vi "xps_panel_DO_connect_to_controller.vi"(8 "error in (no error)":errorcluster, 10 "Login Info":T1={"IP Address"="192.168.0.254", "User"="Administrator", "Password"="Administrator"}, 11 "newport_xps_panel in":refnum<class "newport_xps_panel.lvclass">) -> (0 "error out":errorcluster, 3 "newport_xps_panel out":refnum<class "newport_xps_panel.lvclass">)   [LabVIEW 2015, in "newport_xps_panel.lvclass"]
uses:
  newport_xps_panel.lvclass
  xps_login_info.ctl
  newport_xps/newport_xps.lvclass
  newport_xps/newport_xps.lvclass/newport_xps.ctl
  UI/panel_class/panel.lvclass
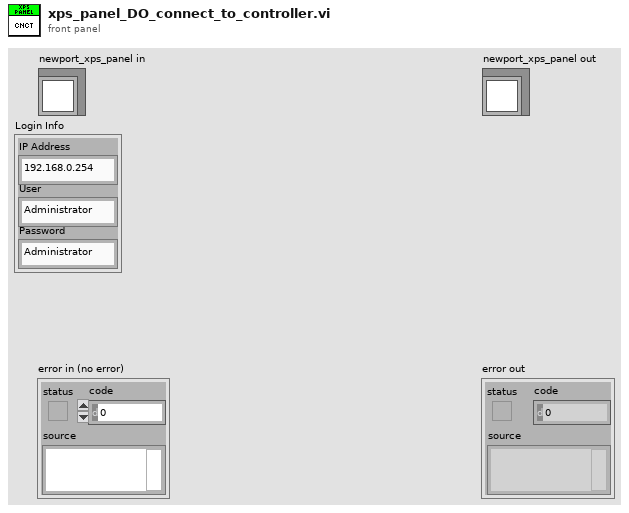
[diagram p1: front panel]
types:
  T1 = typedef "xps_login_info.ctl" = cluster{"IP Address":string, "User":string, "Password":string}
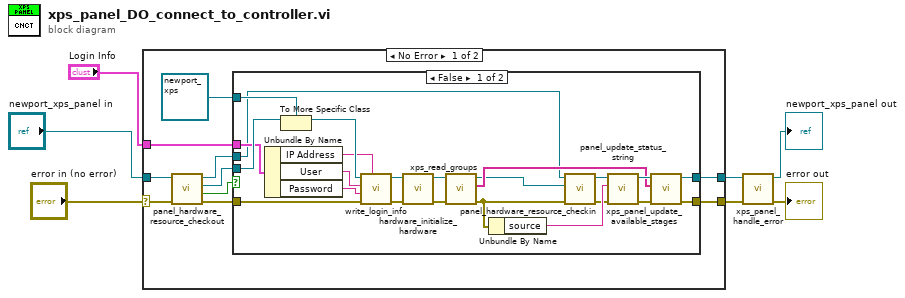
[diagram p0: block diagram]
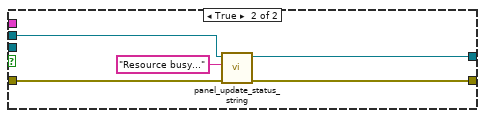
[diagram p2: hidden frame]
diagram:
  n1 = case shown="No Error" "error in (no error)" {
    selector: "error in (no error)" -> [w17 w47]
    tunnel: [w9 w47] -> w4
    tunnel: [w8 w46] -> w2
    tunnel: "newport_xps_panel in" -> [w16 w46]
    tunnel: "Login Info" -> [w10 _]
    frame No Error {
      n2 = call "panel_hardware_resource_checkout.vi"("error in (no error)"=w17, "panel in"=w16) -> ("error out"=w12:errorcluster, "timed out?"=w15:bool, "hardware.lvclass"=w13:refnum<class "hardware.lvclass">, "panel out"=w14:refnum<class "newport_xps_panel.lvclass">)  [unwired: 6 in]
      n3 = case shown="False" w15 {
        tunnel: w14 -> [w21 w42]
        tunnel: w13 -> [w37 _]
        tunnel: w12 -> [w35 w45]
        tunnel: [w20 w44] -> w9
        tunnel: [w22 w41] -> w8
        tunnel: refnum<class "newport_xps.lvclass"> refnum ("newport_xps in") -> [w36 _]
        tunnel: w10 -> [w31 _]
        frame False {
          n4 = Unbundle By Name(w31) -> ("IP Address"=w30:string, "User"=w29:string, "Password"=w28:string)
          n5 = To More Specific Class(target class=w36, reference=w37) -> (specific class reference=w34:refnum<class "newport_xps.lvclass">)  [unwired: 1 in, 1 out]
          n6 = call "write_login_info.vi"("IP address"=w30, "error in (no error)"=w35, "Password"=w28, "User"=w29, "newport_xps in"=w34) -> ("error out"=w32:errorcluster, "newport_xps out"=w33:refnum<class "newport_xps.lvclass">)  [unwired: 5 in]
          n7 = call-dynamic "hardware_initialize_hardware.vi"("error in (no error)"=w32, "newport_xps in"=w33) -> ("error out"=w26:errorcluster, "newport_xps out"=w27:refnum<class "newport_xps.lvclass">)  [unwired: 8 in]
          n8 = call "xps_read_groups.vi"("error in (no error)"=w26, "newport_xps in"=w27) -> ("error out"=w19:errorcluster, "Groups"=w24:string[], "newport_xps out"=w18:refnum<class "newport_xps.lvclass">)  [unwired: 7 in]
          n9 = Unbundle By Name(w19) -> ("source"=w39:string)
          n10 = call "panel_hardware_resource_checkin.vi"("error in (no error)"=w19, "hardware.lvclass"=w18, "panel in"=w21) -> ("error out"=w38:errorcluster, "panel out"=w40:refnum<class "newport_xps_panel.lvclass">)  [unwired: 7 in]
          n11 = call-dynamic "panel_update_status_string.vi"("error in (no error)"=w38, "String"=w39, "newport_xps_panel in"=w40) -> ("error out"=w23:errorcluster, "newport_xps_panel out"=w25:refnum<class "newport_xps_panel.lvclass">)  [unwired: 7 in]
          n12 = call "xps_panel_update_available_stages.vi"("error in (no error)"=w23, "Groups"=w24, "newport_xps_panel in"=w25) -> ("error out"=w20:errorcluster, "newport_xps_panel out"=w22:refnum<class "newport_xps_panel.lvclass">)  [unwired: 7 in]
        }
        frame True {
          n13 = call-dynamic "panel_update_status_string.vi"("error in (no error)"=w45, "String"="Resource busy...", "newport_xps_panel in"=w42) -> ("error out"=w44:errorcluster, "newport_xps_panel out"=w41:refnum<class "newport_xps_panel.lvclass">)  [unwired: 7 in]
        }
      }
    }
    frame Error {
    }
  }
  n14 = call "xps_panel_handle_error.vi"("error in (no error)"=w4, "newport_xps_panel in"=w2) -> ("error out"=→"error out":errorcluster, "newport_xps_panel out"=→"newport_xps_panel out":refnum<class "newport_xps_panel.lvclass">)  [unwired: 8 in]
